vi "initialize_Target_list.vi"(10 "Target File Path":path=path "C:/Weekly Runs/Weekly_runs_General/rt_target.txt", 11 "reference":refnum<vi>) -> (2 "error out":errorcluster)   [LabVIEW 2015]
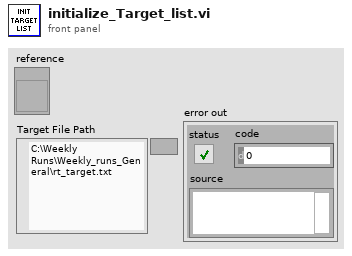
[diagram p1: front panel]
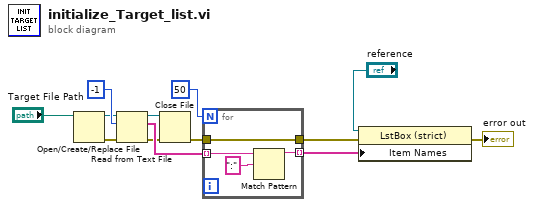
[diagram p0: block diagram]
diagram:
  n1 = Open/Create/Replace File(file path (use dialog)="Target File Path") -> (refnum out=w6:refnum<file>, error out=w7:errorcluster)  [unwired: 5 in, 1 out]
  n2 = Read from Text File(file (use dialog)=w6, count=-1, error in=w7) -> (refnum out=w13:refnum<file>, text=w11:string[], error out=w8:errorcluster)  [unwired: 1 in, 1 out]
  n3 = Close File(refnum=w13, error in=w8) -> (error out=w9:errorcluster)  [unwired: 1 out]
  n4 = for {
    N: 50 -> [_]
    tunnel: [w17] -> w4 mode=indexing
    tunnel: [w16] -> w2
    tunnel: w9 -> [w16]
    tunnel: w11 -> [w14] mode=indexing
    n5 = Match Pattern(string=w14, regular expression=":") -> (before substring=w17:string)  [unwired: 1 in, 3 out]
  }
  n6 = property on="Property Node" class="LstBox (strict)"(reference="reference", error in=w2, "Item Names"=w4) -> (error out=→"error out":errorcluster)  [unwired: 1 out]
